vi "Read User Interface.lvclass.vi"(8 "error in (no error)":errorcluster, 11 "Launch UI Message in":refnum<class "Launch User Interface Msg.lvclass">) -> (0 "error out":errorcluster, 2 "User Interface.lvclass":refnum<class "UI.lvclass">, 3 "Launch UI Message out":refnum<class "Launch User Interface Msg.lvclass">)   [LabVIEW 2017, in "Controller Actor.lvlib" / "Launch User Interface Msg.lvclass"]
uses:
  Launch User Interface Msg.lvclass
  User Interface/UI.lvclass
  Launch User Interface Msg.lvclass/Launch User Interface Msg.ctl
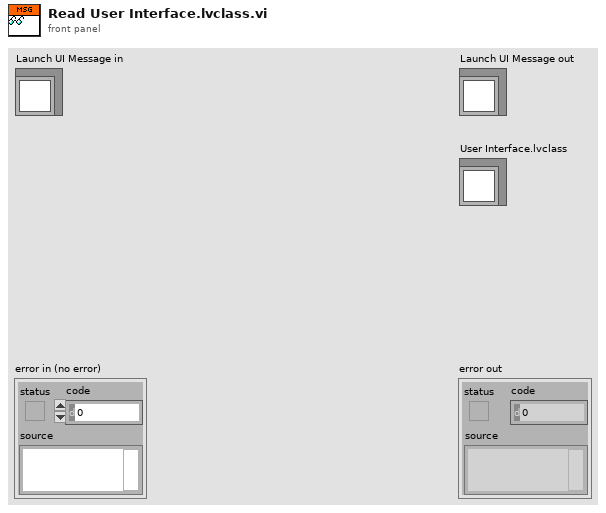
[diagram p1: front panel]
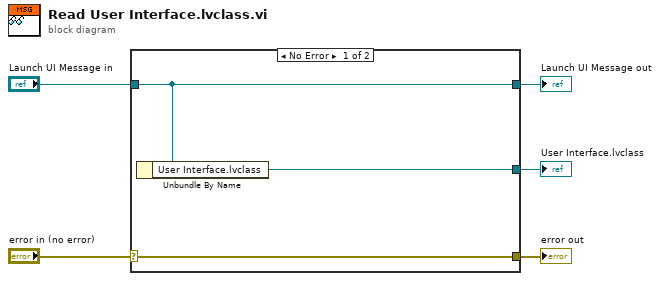
[diagram p0: block diagram]
diagram:
  n1 = case shown="No Error" "error in (no error)" {
    selector: "error in (no error)" -> [w8 w9]
    tunnel: [w8 w9] -> w4
    tunnel: [w7 w10] -> w2
    tunnel: "Launch UI Message in" -> [w7 w10]
    tunnel: [w6 _] -> w1
    frame No Error {
      n2 = Unbundle By Name(w7) -> ("User Interface.lvclass"=w6:refnum<class "UI.lvclass">)
    }
    frame Error {
    }
  }
  "error out" <- w4
  "Launch UI Message out" <- w2
  "User Interface.lvclass" <- w1
